vi "FM_Tx_Template.vi"() -> ()   [LabVIEW 2013]
uses:
  <vilib>/measure/NI_MAPro.lvlib
  <vilib>/Analysis/NI_AALBase.lvlib
  <vilib>/Analysis/baseanly.llb/Quick Scale 1D.vi
  <vilib>/measure/maspectr.llb/FFT Power Spectrum and PSD for 1 Chan.vi
  <vilib>/Analysis/3filter.llb/IIR Filter (DBL).vi
  <vilib>/measure/maspectr.llb/FFT Power Spectrum and PSD for 1 Chan (CDB).vi
  <instrlib>/niUSRP/niUSRP Write Tx Data (CDB WDT).vi
panel:
  out "Frequency Modulated Signal Spectrum":cluster{"f0":dbl, "df":dbl, "magnitude":dbl[]}(graph)
  out "Frequency Modulated Signal":dbl[](graph)
  out "Message Specturm":cluster{"f0":dbl, "df":dbl, "magnitude":dbl[]}(graph)
  out "Message":waveform(dbl)(graph)
  out "Error out":errorcluster
  in  "stop":bool
  in  "Peak Deviation (Hz)":dbl=inf min=inf
  in  "# Tones":i32=3
  in  "Delta Frequency":dbl=1000.0 format="%.2p"
  in  "Start Frequency":dbl=1000.0 format="%.2p"
  in  "Message Length\n(samples)":dbl=200000.0
  in  "Active Antenna":string(combo)="TX1"
  out "Actual Gain (dB)":dbl format="%#_6f"
  in  "Gain (dB)":dbl=20.0 min=0.0 max=31.0 format="%#_6f"
  out "Actual Frequency":dbl=100000.0 format="%#_6p"
  in  "Carrier Frequency":dbl=915100000.0 format="%#_6p"
  out "Actual IQ Rate":dbl=100000.0 format="%#_6p"
  in  "IQ Rate":dbl=200000.0 format="%#_6p"
  in  "Device Names":refnum<k15>="192.168.10.2"
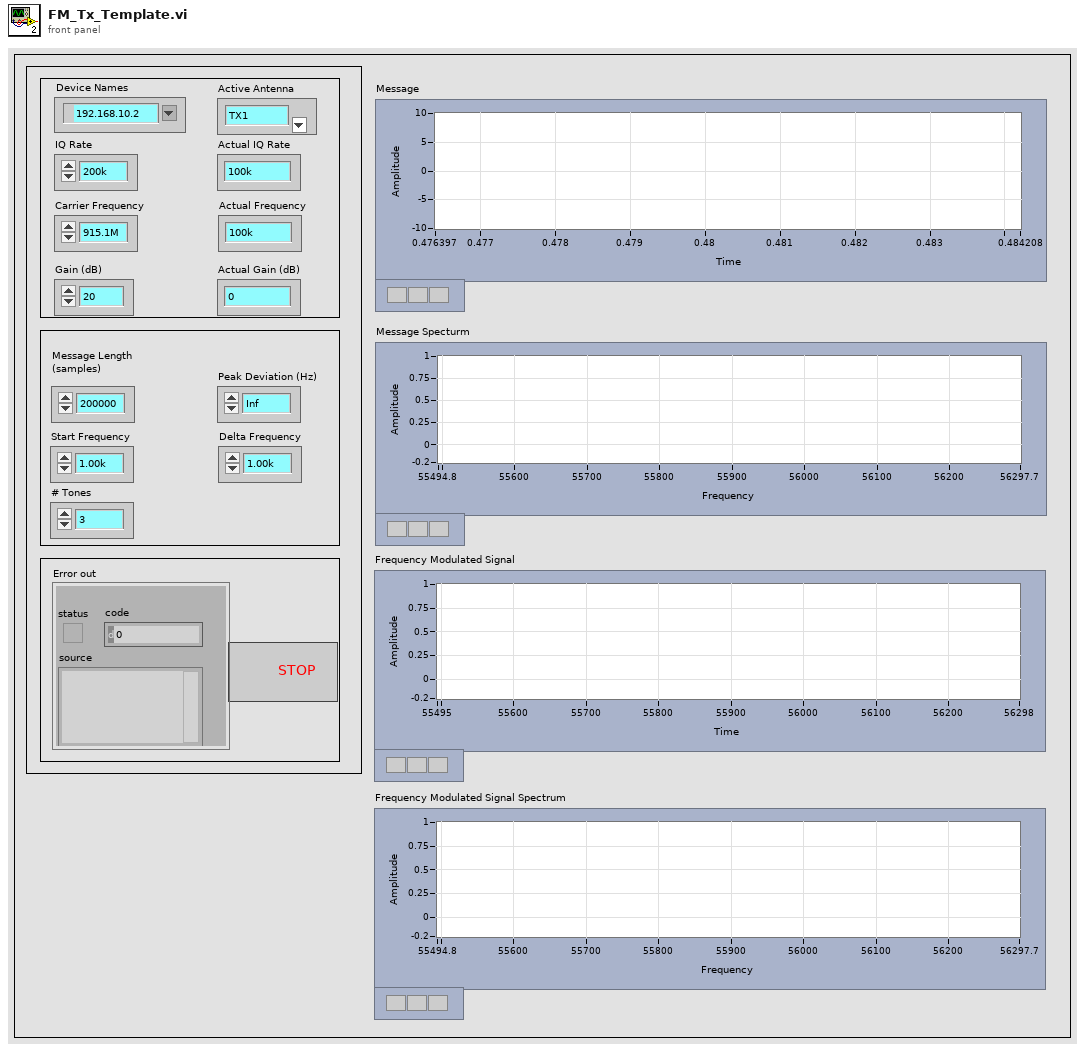
[diagram p1: front panel]
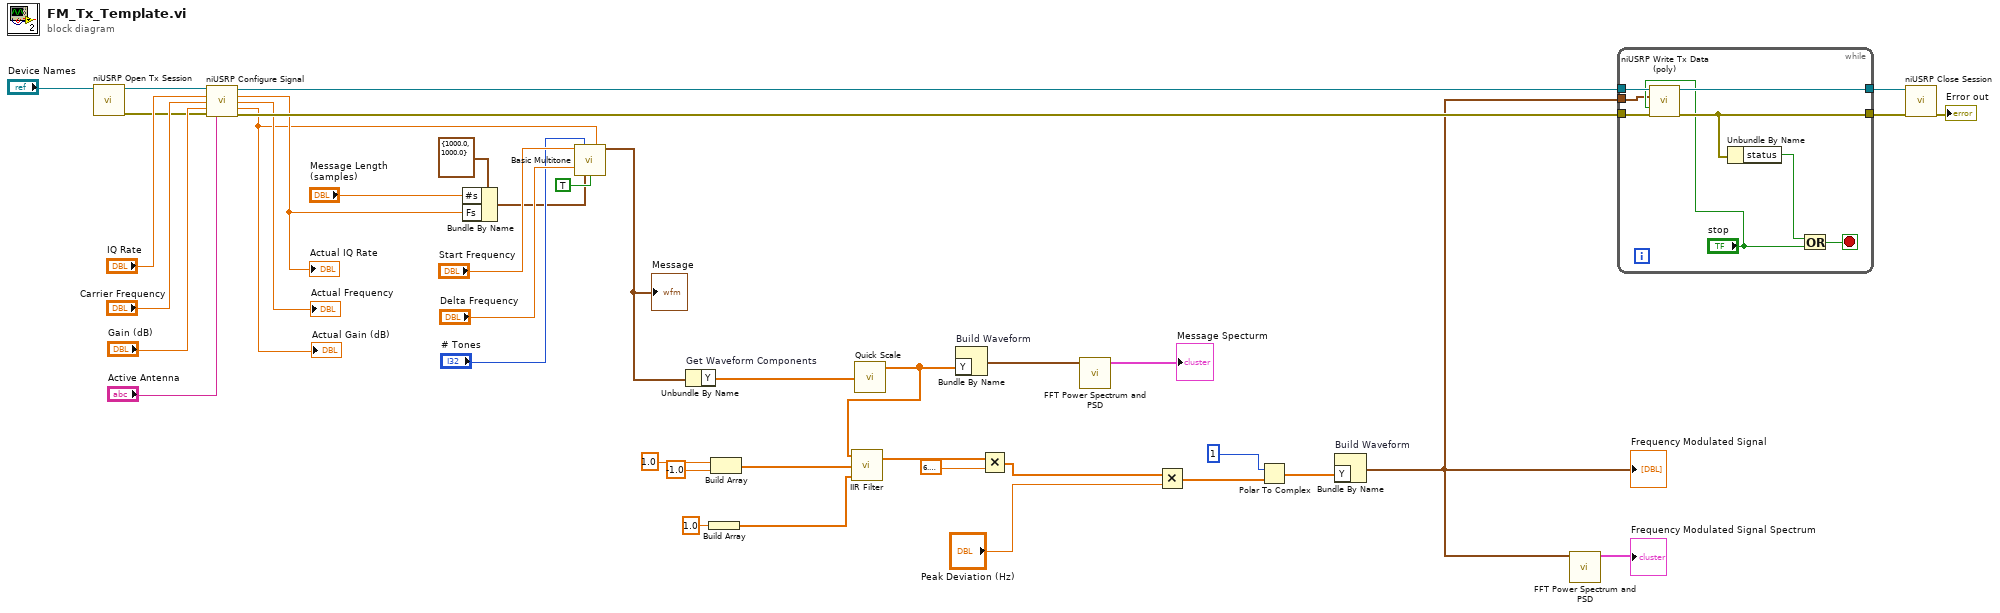
[diagram p0: block diagram]
diagram:
  n1 = call <instrlib>:"niUSRP Open Tx Session.vi"("device names"="Device Names") -> ("session handle out"=w40:refnum<k15>, "error out"=w36:errorcluster)  [unwired: 13 in]
  n2 = call <instrlib>:"niUSRP Configure Signal.vi"("session handle"=w40, "IQ rate"="IQ Rate", "carrier frequency"="Carrier Frequency", "gain"="Gain (dB)", "error in (no error)"=w36, "active antenna"="Active Antenna") -> ("session handle out"=w30:refnum<k15>, "coerced IQ rate"=w22:dbl, "coerced carrier frequency"=→"Actual Frequency":dbl, "coerced gain"=w20:dbl, "error out"=w28:errorcluster)  [unwired: 5 in]
  "Actual IQ Rate" <- w22
  "Actual Gain (dB)" <- w20
  n3 = Bundle By Name(cluster=cluster{"Fs":dbl, "#s":dbl} {"Fs"=1000.0, "#s"=1000.0} ("sampling info"), "#s"="Message Length\n(samples)", "Fs"=w22) -> (w23:cluster{"Fs":dbl, "#s":dbl})
  n4 = call <vilib>:"Basic Multitone.vi"("start frequency"="Start Frequency", "#tones"="# Tones", "amplitude"=w20, "delta frequency"="Delta Frequency", "sampling info"=w23, "coerce frequencies?"=TRUE) -> ("signal out"=w19:waveform(dbl))  [unwired: 6 in, 3 out]
  "Message" <- w19
  n5 = Unbundle By Name "Get Waveform Components"(w19) -> ("Y"=w18:dbl[])
  n6 = Build Array(1.0 ("element")) -> (w10:dbl[])
  n7 = Build Array "Build Array"(1.0, -1.0) -> (w12:dbl[])
  n8 = call-poly <vilib>:"Quick Scale.vi"("X"=w18) -> ("Y[i]=X[i]/Max|X|"=w15:dbl[])  [unwired: 2 out]
  n9 = call-poly <vilib>:"IIR Filter.vi"("Forward Coefficients"=w10, "Reverse Coefficients"=w12, "X"=w15) -> ("Filtered X"=w9:dbl[])  [unwired: 1 in, 1 out]
  n10 = Bundle By Name "Build Waveform"("Y"=w15) -> (w17:waveform(dbl))  [unwired: 1 in]
  n11 = Multiply(x=w9, y=6.283185307179586) -> (x*y=w7:dbl[])
  n12 = call-poly <vilib>:"FFT Power Spectrum and PSD.vi"("time signal"=w17) -> ("Power Spectrum / PSD"=→"Message Specturm":cluster{"f0":dbl, "df":dbl, "magnitude":dbl[]})  [unwired: 7 in, 3 out]
  n13 = Multiply(x=w7, y="Peak Deviation (Hz)") -> (x*y=w5:dbl[])
  n14 = Polar To Complex(1:w5, 2:1) -> (0:w3:cdb[])
  n15 = Bundle By Name "Build Waveform"("Y"=w3) -> (w2:waveform(cdb))  [unwired: 1 in]
  "Frequency Modulated Signal" <- w2
  n16 = call-poly <vilib>:"FFT Power Spectrum and PSD.vi"("time signal"=w2) -> ("Power Spectrum / PSD"=→"Frequency Modulated Signal Spectrum":cluster{"f0":dbl, "df":dbl, "magnitude":dbl[]})  [unwired: 7 in, 3 out]
  n17 = while {
    tunnel: w30 -> [w49]
    tunnel: [w48] -> w29
    tunnel: w28 -> [w47]
    tunnel: [w46] -> w25
    tunnel: w2 -> [w42]
    stop <- w44 stop-if-true
    n18 = call-poly <instrlib>:"niUSRP Write Tx Data (poly).vi"("session handle"=w49, "data"=w42, "end of data?"="stop", "error in (no error)"=w47) -> ("session handle out"=w48:refnum<k15>, "error out"=w46:errorcluster)  [unwired: 10 in]
    n19 = Unbundle By Name(w46) -> ("status"=w45:bool)
    n20 = Or(x=w45, y="stop") -> (x .or. y?=w44:bool)
  }
  n21 = call <instrlib>:"niUSRP Close Session.vi"("session handle"=w29, "error in (no error)"=w25) -> ("error out"=→"Error out":errorcluster)  [unwired: 13 in]
